vi "IMAQ FPGA Camera Link Data to Pixels.vi"   [LabVIEW 2020]
doc: "Reads the bits from the Camera Link data ports and organizes the bits into pixels for the requested tap configuration."
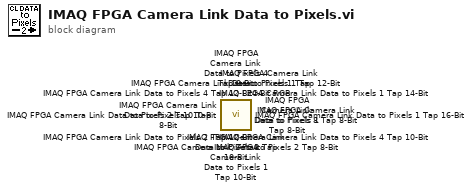
[diagram p0: block diagram]
diagram:
  n1 = call <vilib>:"IMAQ FPGA Camera Link Data to Pixels 8 Tap 10-Bit.vi"() -> ()  [unwired: 1 in, 1 out]
  n2 = call <vilib>:"IMAQ FPGA Camera Link Data to Pixels 1 Tap 24-Bit RGB.vi"() -> ()  [unwired: 1 in, 1 out]
  n3 = call <vilib>:"IMAQ FPGA Camera Link Data to Pixels 10 Tap 8-Bit.vi"() -> ()  [unwired: 1 in, 1 out]
  n4 = call <vilib>:"IMAQ FPGA Camera Link Data to Pixels 8 Tap 8-Bit.vi"() -> ()  [unwired: 1 in, 1 out]
  n5 = call <vilib>:"IMAQ FPGA Camera Link Data to Pixels 4 Tap 12-Bit.vi"() -> ()  [unwired: 1 in, 1 out]
  n6 = call <vilib>:"IMAQ FPGA Camera Link Data to Pixels 4 Tap 10-Bit.vi"() -> ()  [unwired: 1 in, 1 out]
  n7 = call <vilib>:"IMAQ FPGA Camera Link Data to Pixels 4 Tap 8-Bit.vi"() -> ()  [unwired: 1 in, 1 out]
  n8 = call <vilib>:"IMAQ FPGA Camera Link Data to Pixels 2 Tap 12-Bit.vi"() -> ()  [unwired: 1 in, 1 out]
  n9 = call <vilib>:"IMAQ FPGA Camera Link Data to Pixels 2 Tap 10-Bit.vi"() -> ()  [unwired: 1 in, 1 out]
  n10 = call <vilib>:"IMAQ FPGA Camera Link Data to Pixels 2 Tap 8-Bit.vi"() -> ()  [unwired: 1 in, 1 out]
  n11 = call <vilib>:"IMAQ FPGA Camera Link Data to Pixels 1 Tap 16-Bit.vi"() -> ()  [unwired: 1 in, 1 out]
  n12 = call <vilib>:"IMAQ FPGA Camera Link Data to Pixels 1 Tap 14-Bit.vi"() -> ()  [unwired: 1 in, 1 out]
  n13 = call <vilib>:"IMAQ FPGA Camera Link Data to Pixels 1 Tap 12-Bit.vi"() -> ()  [unwired: 1 in, 1 out]
  n14 = call <vilib>:"IMAQ FPGA Camera Link Data to Pixels 1 Tap 10-Bit.vi"() -> ()  [unwired: 1 in, 1 out]
  n15 = call <vilib>:"IMAQ FPGA Camera Link Data to Pixels 1 Tap 8-Bit.vi"() -> ()  [unwired: 1 in, 1 out]
